vi "Write First Time.vi"(8 "error in (no error)":errorcluster, 10 "First Time":dbl, 11 "Readout Charact in":refnum<class "Readout Charact.lvclass">) -> (0 "error out":errorcluster, 3 "Readout Charact out":refnum<class "Readout Charact.lvclass">)   [LabVIEW 2018, in "Readout Charact.lvclass"]
uses:
  Readout Charact.lvclass
  Readout Charact.lvclass/Readout Charact.ctl
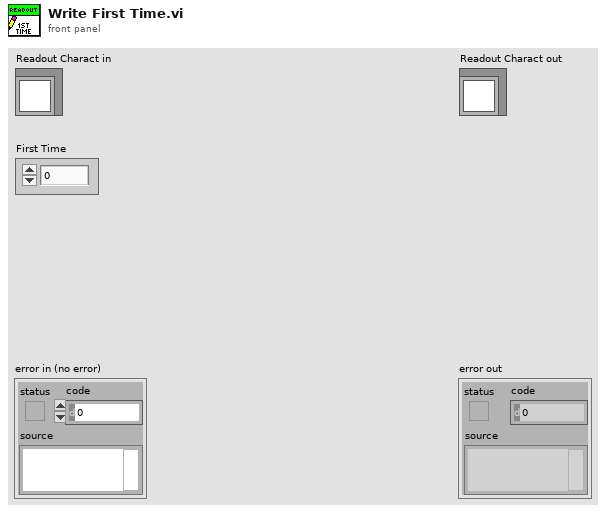
[diagram p1: front panel]
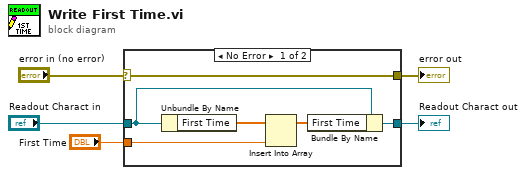
[diagram p0: block diagram]
diagram:
  n1 = case shown="No Error" "error in (no error)" {
    selector: "error in (no error)" -> [w11 w12]
    tunnel: [w11 w12] -> w4
    tunnel: [w6 w13] -> w2
    tunnel: "Readout Charact in" -> [w7 w13]
    tunnel: "First Time" -> [w8 _]
    frame No Error {
      n2 = Unbundle By Name(w7) -> ("First Time"=w10:dbl[])
      n3 = Insert Into Array(array=w10, new element=w8) -> (w9:dbl[])  [unwired: 1 in]
      n4 = Bundle By Name(cluster=w7, "First Time"=w9) -> (w6:refnum<class "Readout Charact.lvclass">)
    }
    frame Error {
    }
  }
  "error out" <- w4
  "Readout Charact out" <- w2
